vi "init_MAG5173.vi"(0 "iIndex":u32, 5 "I2C speed":T9(ring)=enum."standard (100kHz)", 7 "X, Y Range - Low / High":T3(ring)=enum."±80mT (TMAG5173A1) or ±266mT (TMAG5173A2)", 9 "Z Range - Low / High":T3(ring)=enum."±80mT (TMAG5173A1) or ±266mT (TMAG5173A2)") -> (4 "oIndex":u32, 6 "DeviceID":u8 format="%02x", 8 "X_Y_Range":dbl, 10 "Z_Range":dbl, 15 "error out":errorcluster)   [LabVIEW 2011]
panel:
  out "Sensor_Config_1":T1 {"MAG_Ch_EN" format="%x"}
  out "Sensor_Config_2":T2
  in  "magnetic Axes":T4(ring)=enum."X, Y, Z channel enabled"
  out "Device_Config_1":T5
  in  "Hardware Average":T6(ring)=enum."32x average, 0.4-kSPS (3-axes) or 1.2-kSPS (1 axis)"
  out "Device_Config_2":T7
  out "Sensor Variante":T8(ring)
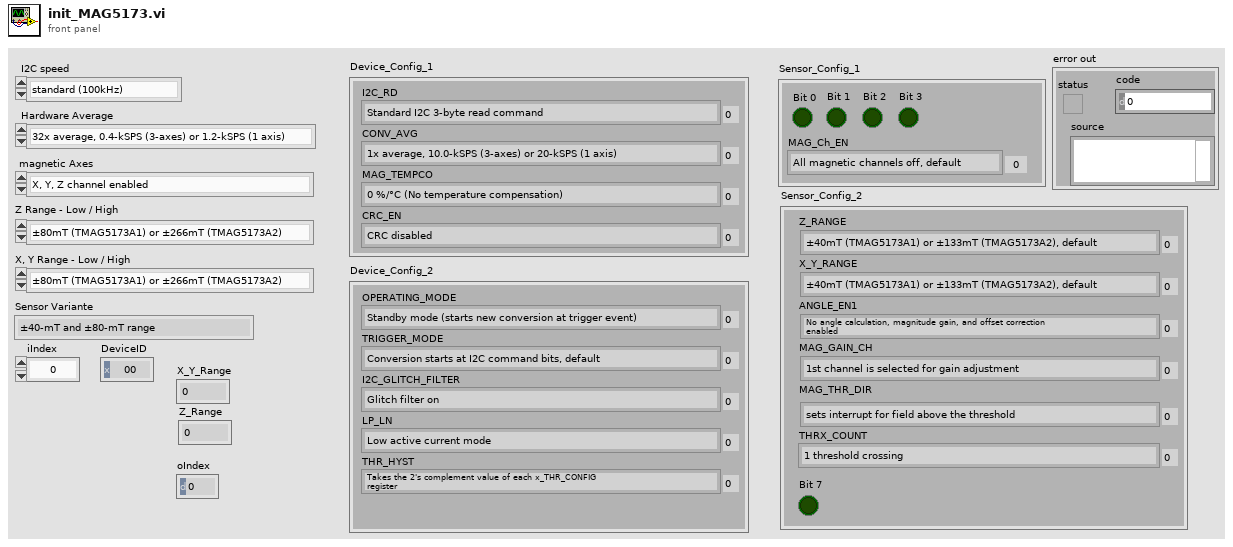
[diagram p1: front panel]
types:
  T1 = cluster{"Bit 0":bool, "Bit 1":bool, "Bit 2":bool, "Bit 3":bool, "MAG_Ch_EN":enum8{"All magnetic channels off, default", "X channel enabled", "Y channel enabled", "X, Y channel enabled", "Z channel enabled", "Z, X channel enabled", "Y, Z channel enabled", "X, Y, Z channel enabled", "XYX channel enabled", "YXY channel enabled", "YZY channel enabled", "XZX channel enabled", "X, Y, Z with positive AFE diagnostic check", "X, Y, Z with negative AFE diagnostic check", "Hall resistance check + ADC check", "Hall offset check +ADC check"}}
  T2 = cluster{"Z_RANGE":enum8{"±40mT (TMAG5173A1) or ±133mT (TMAG5173A2), default", "±80mT (TMAG5173A1) or ±266mT (TMAG5173A2)"}, "X_Y_RANGE":enum8{"±40mT (TMAG5173A1) or ±133mT (TMAG5173A2), default", "±80mT (TMAG5173A1) or ±266mT (TMAG5173A2)"}, "ANGLE_EN1":enum8{"No angle calculation, magnitude gain, and offset correction\nenabled", "X 1st, Y 2nd", "Y 1st, Z 2nd", "X 1st, Z 2nd"}, "MAG_GAIN_CH":enum8{"1st channel is selected for gain adjustment", "2nd channel is selected for gain adjustment"}, "MAG_THR_DIR":enum8{"sets interrupt for field above the threshold", "sets interrupt for field below the threshold"}, "THRX_COUNT":enum8{"1 threshold crossing", "4 threshold crossing"}, "Bit 7":bool}
  T3 = enum8{"±40mT (TMAG5173A1) or ±133mT (TMAG5173A2), default", "±80mT (TMAG5173A1) or ±266mT (TMAG5173A2)"}
  T4 = enum8{"All magnetic channels off, default", "X channel enabled", "Y channel enabled", "X, Y channel enabled", "Z channel enabled", "Z, X channel enabled", "Y, Z channel enabled", "X, Y, Z channel enabled", "XYX channel enabled", "YXY channel enabled", "YZY channel enabled", "XZX channel enabled", "X, Y, Z with positive AFE diagnostic check", "X, Y, Z with negative AFE diagnostic check", "Hall resistance check + ADC check", "Hall offset check +ADC check"}
  T5 = cluster{"I2C_RD":enum8{"Standard I2C 3-byte read command", "1-byte I2C read command for 16bit sensor data and conversion\nstatus", "1-byte I2C read command for 8 bit sensor MSB data and\nconversion status", "Reserved"}, "CONV_AVG":enum8{"1x average, 10.0-kSPS (3-axes) or 20-kSPS (1 axis)", "2x average, 5.7-kSPS (3-axes) or 13.3-kSPS (1 axis)", "4x average, 3.1-kSPS (3-axes) or 8.0-kSPS (1 axis)", "8x average, 1.6-kSPS (3-axes) or 4.4-kSPS (1 axis)", "16x average, 0.8-kSPS (3-axes) or 2.4-kSPS (1 axis)", "32x average, 0.4-kSPS (3-axes) or 1.2-kSPS (1 axis)"}, "MAG_TEMPCO":enum8{"0 %/°C (No temperature compensation)", "0.12 %/°C (NdBFe)", "0.03 %/°C (SmCo)", "0.20 %/°C (Ceramic)"}, "CRC_EN":enum8{"CRC disabled", "CRC enabled"}}
  T6 = enum8{"1x average, 10.0-kSPS (3-axes) or 20-kSPS (1 axis)", "2x average, 5.7-kSPS (3-axes) or 13.3-kSPS (1 axis)", "4x average, 3.1-kSPS (3-axes) or 8.0-kSPS (1 axis)", "8x average, 1.6-kSPS (3-axes) or 4.4-kSPS (1 axis)", "16x average, 0.8-kSPS (3-axes) or 2.4-kSPS (1 axis)", "32x average, 0.4-kSPS (3-axes) or 1.2-kSPS (1 axis)"}
  T7 = cluster{"OPERATING_MODE":enum8{"Standby mode (starts new conversion at trigger event)", "Sleep mode", "Continuous measure mode", "Reserved"}, "TRIGGER_MODE":enum8{"Conversion starts at I2C command bits, default", "Conversion starts through a trigger signal at the INT pin"}, "I2C_GLITCH_FILTER":enum8{"Glitch filter on", "Glitch filter off"}, "LP_LN":enum8{"Low active current mode", "Low noise mode"}, "THR_HYST":enum8{"Takes the 2's complement value of each x_THR_CONFIG\nregister", "Takes the 7 LSB bits of the x_THR_CONFIG register", "8 LSB threshold band, 12 bit resolution", "16 LSB threshold band, 12 bit resolution", "32 LSB threshold, band 12 bit resolution", "64 LSB threshold band, 12 bit resolution", "128 LSB threshold band, 12 bit resolution", "256 LSB threshold band, 12 bit resolution"}}
  T8 = enum8{"±40-mT and ±80-mT range", "Reserved", "±133-mT and ±266-mT range", "Reserved."}
  T9 = enum32{"low speed (20kHz)", "standard (100kHz)", "fast (400kHz)", "high speed (750kHz)"}
  T10 = enum8{"Low active current mode", "Low noise mode"}
  T11 = enum8{"Standby mode (starts new conversion at trigger event)", "Sleep mode", "Continuous measure mode", "Reserved"}
  T12 = cluster{"T_CH_EN":enum8{"Temp channel disabled", "Temp channel enabled"}, "T_THR_CONFIG":u8}
  T13 = enum8{"Standard I2C 3-byte read command", "1-byte I2C read command for 16bit sensor data and conversion\nstatus", "1-byte I2C read command for 8 bit sensor MSB data and\nconversion status", "Reserved"}
  T14 = cluster{"VER":enum8{"±40-mT and ±80-mT range", "Reserved", "±133-mT and ±266-mT range", "Reserved."}, "Bit2":bool, "Bit3":bool, "Bit4":bool, "Bit5":bool, "Bit6":bool, "Bit7":bool}
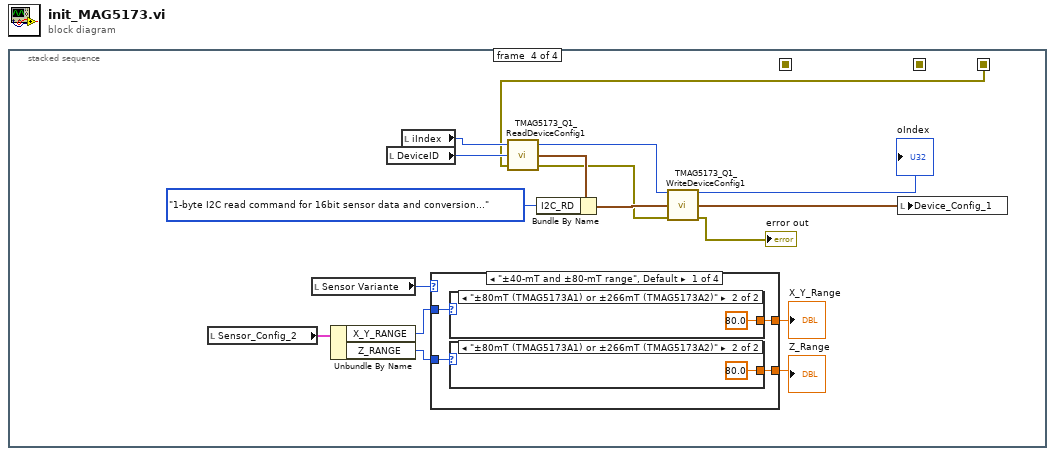
[diagram p0: block diagram]
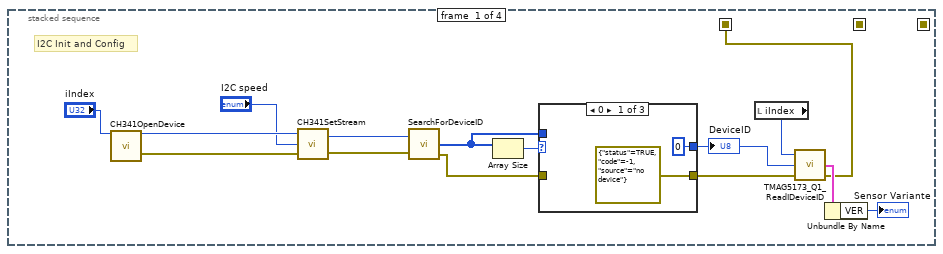
[diagram p2: hidden frame]
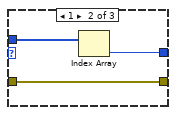
[diagram p3: hidden frame]
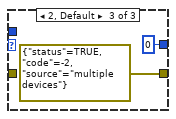
[diagram p4: hidden frame]
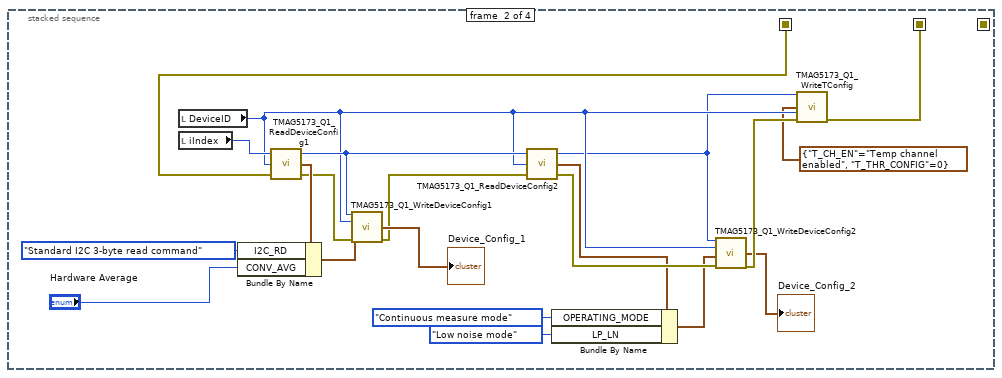
[diagram p5: hidden frame]
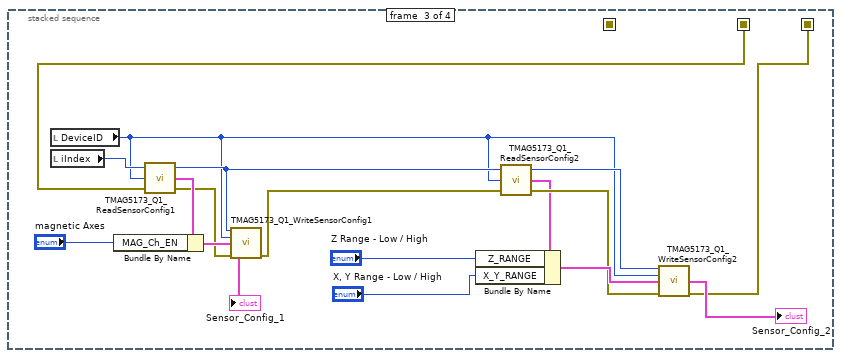
[diagram p6: hidden frame]
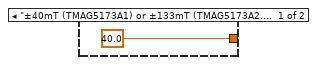
[diagram p7: hidden frame]
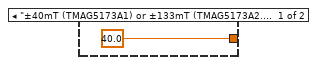
[diagram p8: hidden frame]
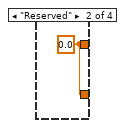
[diagram p9: hidden frame]
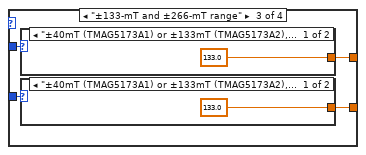
[diagram p10: hidden frame]
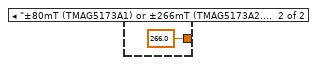
[diagram p11: hidden frame]
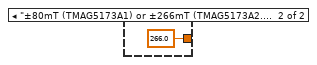
[diagram p12: hidden frame]
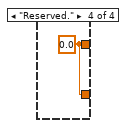
[diagram p13: hidden frame]
diagram:
  n1 = stacked-sequence {
    seq-local: [w2 _ _ _] -> [_ w30 _ _]
    seq-local: [_ w29 _ _] -> [_ _ w48 _]
    seq-local: [_ _ w49 _] -> [_ _ _ w69]
    frame #0 {
      # "I2C Init and Config"
      n2 = call <userlib>:"CH341OpenDevice.vi"("iIndex"="iIndex") -> ("oIndex"=w14:u32, "error out"=w13:errorcluster)  [unwired: 12 in, 1 out]
      n3 = call <userlib>:"CH341SetStream.vi"("error in (no error)"=w13, "speed"="I2C speed", "iIndex"=w14) -> ("error out"=w11:errorcluster, "oIndex"=w12:u32)
      n4 = call <userlib>:"SearchForDeviceID.vi"("error in (no error)"=w11, "iIndex"=w12) -> ("error out"=w8:errorcluster, "Device List"=w9:u8[])  [unwired: 1 out]
      n5 = Array Size(array=w9) -> (size(s)=w10:i32)
      n6 = case shown="0" w10 {
        tunnel: w9 -> [_ w19 _]
        tunnel: [errorcluster {"status"=TRUE, "code"=-1, "source"="no device"} ("error in (no error)") w20 errorcluster {"status"=TRUE, "code"=-2, "source"="multiple devices"} ("error in (no error)")] -> w7
        tunnel: w8 -> [_ w20 _]
        tunnel: [u8 0 ("t") w18 u8 0 ("t")] -> w3
        frame 0 {
        }
        frame 1 {
          n7 = Index Array(array=w19) -> (element=w18:u8)  [unwired: 1 in]
        }
        frame 2, Default {
        }
      }
      "DeviceID" <- w3
      n8 = local read "iIndex"() -> (w6:u32)
      n9 = call <userlib>:"TMAG5173_Q1_ReadIDeviceID.vi"("error in (no error)"=w7, "DeviceID"=w3, "iIndex"=w6) -> ("error out"=w2:errorcluster, "Device_ID"=w5:T14)  [unwired: 1 out]
      n10 = Unbundle By Name(w5) -> ("VER"=→"Sensor Variante":T8)
    }
    frame #1 {
      n11 = local read "DeviceID"() -> (w34:u8)
      n12 = local read "iIndex"() -> (w43:u32)
      n13 = call <userlib>:"TMAG5173_Q1_ReadDeviceConfig1.vi"("error in (no error)"=w30, "DeviceID"=w34, "iIndex"=w43) -> ("error out"=w37:errorcluster, "Device_Config_1"=w40:T5, "oIndex"=w38:u32)
      n14 = Bundle By Name(cluster=w40, "I2C_RD"=T13."Standard I2C 3-byte read command", "CONV_AVG"="Hardware Average") -> (w39:T5)
      n15 = call <userlib>:"TMAG5173_Q1_WriteDeviceConfig1.vi"("iIndex"=w38, "DeviceID"=w34, "Device_Config_1"=w39, "error in (no error)"=w37) -> ("Device_Config_1 out"=→"Device_Config_1":T5, "error out"=w36:errorcluster)  [unwired: 9 in, 1 out]
      n16 = call <userlib>:"TMAG5173_Q1_ReadDeviceConfig2.vi"("error in (no error)"=w36, "DeviceID"=w34, "iIndex"=w38) -> ("error out"=w42:errorcluster, "Device_Config_2"=w26:T7, "oIndex"=w33:u32)
      n17 = Bundle By Name(cluster=w26, "OPERATING_MODE"=T11."Continuous measure mode", "LP_LN"=T10."Low noise mode") -> (w25:T7)
      n18 = call <userlib>:"TMAG5173_Q1_WriteDeviceConfig2.vi"("iIndex"=w33, "DeviceID"=w34, "Device_Config_2"=w25, "error in (no error)"=w42) -> ("Device_Config_2 out"=→"Device_Config_2":T7, "error out"=w32:errorcluster)  [unwired: 9 in, 1 out]
      n19 = call <userlib>:"TMAG5173_Q1_WriteTConfig.vi"("iIndex"=w33, "DeviceID"=w34, "T_Config"=T12 {"T_CH_EN"=enum."Temp channel enabled", "T_THR_CONFIG"=0}, "error in (no error)"=w32) -> ("error out"=w29:errorcluster)  [unwired: 9 in, 2 out]
    }
    frame #2 {
      n20 = local read "DeviceID"() -> (w51:u8)
      n21 = local read "iIndex"() -> (w61:u32)
      n22 = call <userlib>:"TMAG5173_Q1_ReadSensorConfig1.vi"("error in (no error)"=w48, "iDevice"=w51, "iIndex"=w61) -> ("error out"=w57:errorcluster, "Sensor_Config_1"=w59:T1, "oIndes"=w55:u32)
      n23 = Bundle By Name(cluster=w59, "MAG_Ch_EN"="magnetic Axes") -> (w58:T1)
      n24 = call <userlib>:"TMAG5173_Q1_WriteSensorConfig1.vi"("iIndex"=w55, "DeviceID"=w51, "Sensor_Config_1"=w58, "error in (no error)"=w57) -> ("Sensor_Config_1 out"=→"Sensor_Config_1":T1, "error out"=w56:errorcluster)  [unwired: 9 in, 1 out]
      n25 = call <userlib>:"TMAG5173_Q1_ReadSensorConfig2.vi"("error in (no error)"=w56, "DeviceID"=w51, "iIndex"=w55) -> ("error out"=w50:errorcluster, "Sensor_Config_2"=w47:T2, "oIndex"=w52:u32)
      n26 = Bundle By Name(cluster=w47, "Z_RANGE"="Z Range - Low / High", "X_Y_RANGE"="X, Y Range - Low / High") -> (w53:T2)
      n27 = call <userlib>:"TMAG5173_Q1_WriteSensorConfig2.vi"("iIndex"=w52, "DeviceID"=w51, "Sensor_Config_2"=w53, "error in (no error)"=w50) -> ("Sensor_Config_2 out"=→"Sensor_Config_2":T2, "error out"=w49:errorcluster)  [unwired: 9 in, 1 out]
    }
    frame #3 {
      n28 = local read "Sensor_Config_2"() -> (w67:T2)
      n29 = local read "Sensor Variante"() -> (w68:T8)
      n30 = Unbundle By Name(w67) -> ("X_Y_RANGE"=w66:T3, "Z_RANGE"=w65:T3)
      n31 = local read "DeviceID"() -> (w72:u8)
      n32 = local read "iIndex"() -> (w73:u32)
      n33 = case shown="\"±40-mT and ±80-mT range\", Default" w68 {
        tunnel: w66 -> [w82 _ w89 _]
        tunnel: w65 -> [w80 _ w88 _]
        tunnel: [w81 w87 w91 w96] -> w64
        tunnel: [w79 w87 w90 w96] -> w63
        frame "±40-mT and ±80-mT range", Default {
          n34 = case shown="\"±80mT (TMAG5173A1) or ±266mT (TMAG5173A2)\"" w82 {
            tunnel: [40.0 80.0] -> w81
            frame "±40mT (TMAG5173A1) or ±133mT (TMAG5173A2), default", Default {
            }
            frame "±80mT (TMAG5173A1) or ±266mT (TMAG5173A2)" {
            }
          }
          n35 = case shown="\"±80mT (TMAG5173A1) or ±266mT (TMAG5173A2)\"" w80 {
            tunnel: [40.0 80.0] -> w79
            frame "±40mT (TMAG5173A1) or ±133mT (TMAG5173A2), default", Default {
            }
            frame "±80mT (TMAG5173A1) or ±266mT (TMAG5173A2)" {
            }
          }
        }
        frame "Reserved" {
          w87 = 0.0
        }
        frame "±133-mT and ±266-mT range" {
          n36 = case shown="\"±40mT (TMAG5173A1) or ±133mT (TMAG5173A2), default\", Default" w89 {
            tunnel: [133.0 266.0] -> w91
            frame "±40mT (TMAG5173A1) or ±133mT (TMAG5173A2), default", Default {
            }
            frame "±80mT (TMAG5173A1) or ±266mT (TMAG5173A2)" {
            }
          }
          n37 = case shown="\"±40mT (TMAG5173A1) or ±133mT (TMAG5173A2), default\", Default" w88 {
            tunnel: [133.0 266.0] -> w90
            frame "±40mT (TMAG5173A1) or ±133mT (TMAG5173A2), default", Default {
            }
            frame "±80mT (TMAG5173A1) or ±266mT (TMAG5173A2)" {
            }
          }
        }
        frame "Reserved." {
          w96 = 0.0
        }
      }
      "X_Y_Range" <- w64
      "Z_Range" <- w63
      n38 = call <userlib>:"TMAG5173_Q1_ReadDeviceConfig1.vi"("error in (no error)"=w69, "DeviceID"=w72, "iIndex"=w73) -> ("error out"=w74:errorcluster, "Device_Config_1"=w78:T5, "oIndex"=w75:u32)
      n39 = Bundle By Name(cluster=w78, "I2C_RD"=T13."1-byte I2C read command for 16bit sensor data and conversion\nstatus") -> (w77:T5)
      n40 = call <userlib>:"TMAG5173_Q1_WriteDeviceConfig1.vi"("iIndex"=w75, "Device_Config_1"=w77, "error in (no error)"=w74) -> ("oIndex"=→"oIndex":u32, "Device_Config_1 out"=w70:T5, "error out"=→"error out":errorcluster)  [unwired: 10 in]
      n41 = local write "Device_Config_1"(w70) -> ()
    }
  }
